vi "UDP Stream Reader.vi"() -> ()   [LabVIEW 2017]
uses:
  <vilib>/ptbypt/NI_PtbyPt.lvlib
panel:
  out "Chart":dbl(graph)=869191.9467676225
  out "Average Rate":dbl=904314.6721829617 format="%0.1pbytes/second"
  out "UDP Chunks Dropped":bool
  out "Total Heartbeats":i32=21
  out "Data Length":i32=17515
  in  "Stop":bool
  in  "Stream Source IP Address":string="localhost"
  # "UDP Streamer.vi must be running first!"
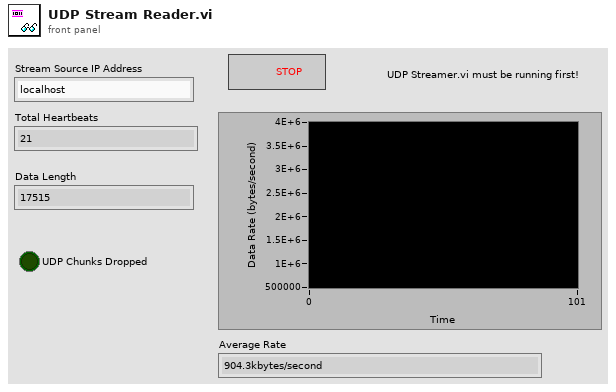
[diagram p1: front panel]
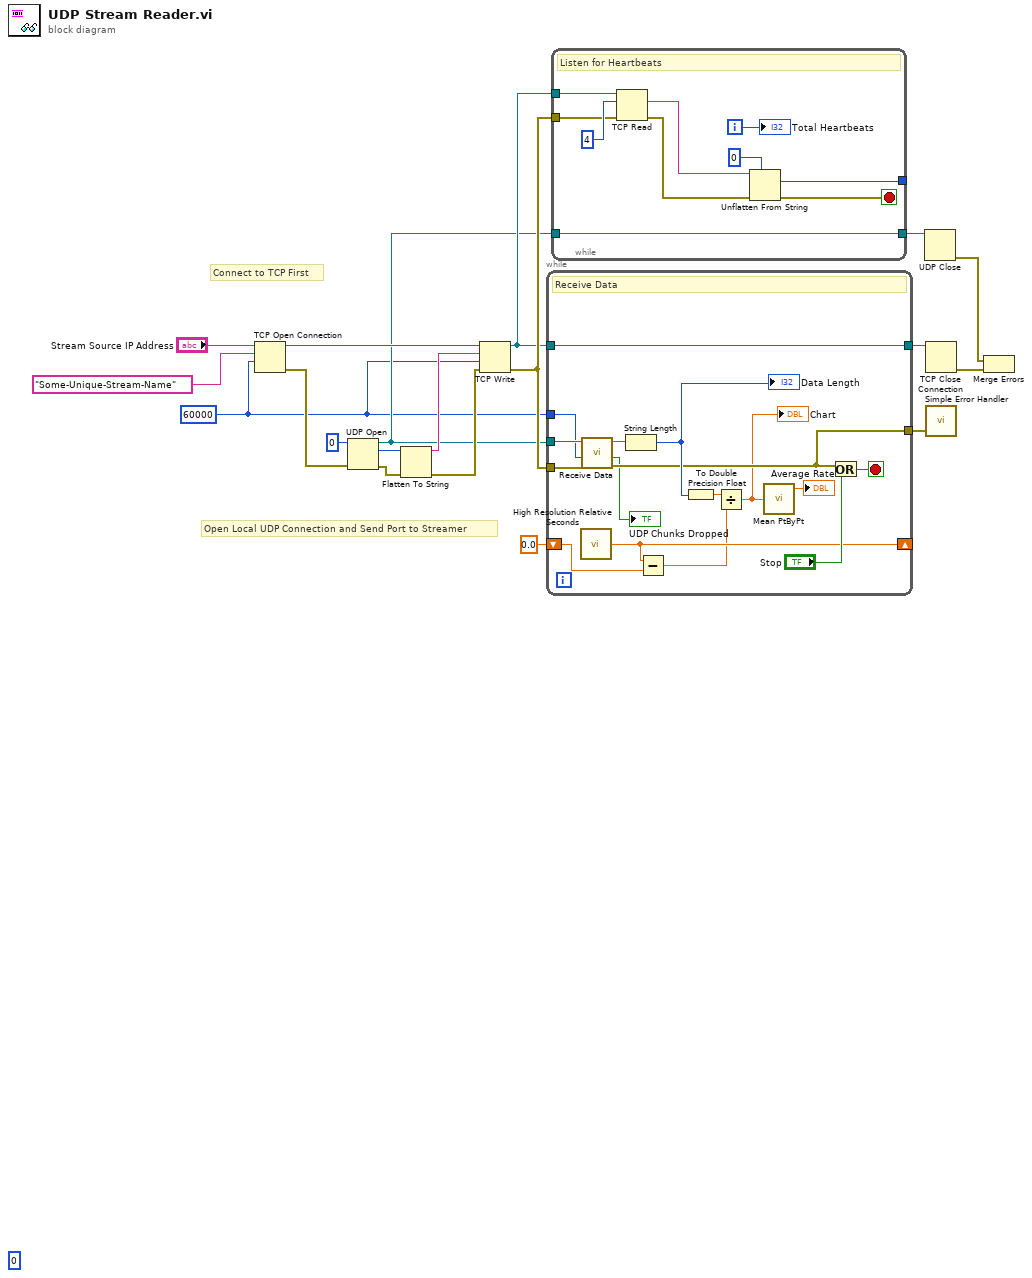
[diagram p0: block diagram]
diagram:
  w1 = 60000 ("timeout ms (60000)")
  (unwired) u32 0
  # "Open Local UDP Connection and Send Port to Streamer"
  # "Connect to TCP First"
  n1 = TCP Open Connection(address="Stream Source IP Address", remote port or service name="Some-Unique-Stream-Name", timeout ms (60000)=w1) -> (connection ID=w13:refnum<k5>, error out=w16:errorcluster)  [unwired: 2 in]
  n2 = UDP Open(8:w16, 11:u16 0 ("port")) -> (port=w7:refnum<k16>, 0:w15:errorcluster, 2:w14:u16)  [unwired: 3 in]
  n3 = Flatten To String(anything=w14, error in (no error)=w15) -> (data string=w11:string, error out=w12:errorcluster)  [unwired: 2 in, 1 out]
  n4 = TCP Write(connection ID=w13, data in=w11, error in (no error)=w12, 9:w1) -> (connection ID out=w8:refnum<k5>, error out=w10:errorcluster)  [unwired: 1 out]
  n5 = while {
    tunnel: w10 -> [w34]
    tunnel: [w33] -> w9
    tunnel: w8 -> [w33]
    tunnel: w7 -> [w35]
    shift-right: [w29] -> _
    shift-left: 0.0 ("relative seconds") -> [w30]
    tunnel: [w25] -> w2
    tunnel: w1 -> [w24]
    stop <- w31 stop-if-true
    # "Receive Data"
    n6 = call <vilib>:"High Resolution Relative Seconds.vi"() -> ("relative seconds"=w29:dbl)
    n7 = call "Receive Data.vi"("error in (no error)"=w34, "timeout ms (25000)"=w24, "UDP Network Connection in"=w35) -> ("error out"=w25:errorcluster, "Chunks Dropped"=→"UDP Chunks Dropped":bool, "Data"=w23:string)  [unwired: 6 in]
    n8 = String Length(string=w23) -> (length=w26:i32)
    "Data Length" <- w26
    n9 = Subtract(x=w29, y=w30) -> (x-y=w28:dbl)
    n10 = To Double Precision Float(number=w26) -> (double precision float=w27:dbl)
    n11 = Divide(x=w27, y=w28) -> (x/y=w20:dbl)
    "Chart" <- w20
    n12 = call <vilib>:"Mean PtByPt.vi"("x"=w20) -> ("mean"=→"Average Rate":dbl)  [unwired: 3 in, 1 out]
    n13 = Or(x=w25, y="Stop") -> (x .or. y?=w31:bool)
  }
  n14 = while {
    tunnel: w10 -> [w39]
    tunnel: w8 -> [w38]
    tunnel: w7 -> [w37]
    tunnel: [w37] -> w6
    tunnel: [w36] -> _
    i -> [w45]
    stop <- w40 stop-if-true
    # "Listen for Heartbeats"
    n15 = TCP Read(connection ID=w38, bytes to read=4, error in (no error)=w39) -> (data out=w43:string, error out=w41:errorcluster)  [unwired: 2 in, 1 out]
    n16 = Unflatten From String(type=0 ("bytes to read"), binary string=w43, error in (no error)=w41) -> (value=w36:i32, error out=w40:errorcluster)  [unwired: 2 in, 1 out]
    "Total Heartbeats" <- w45
  }
  n17 = UDP Close(connection ID=w6) -> (error out=w4:errorcluster)  [unwired: 1 in, 1 out]
  n18 = TCP Close Connection(connection ID=w9) -> (error out=w5:errorcluster)  [unwired: 2 in, 1 out]
  n19 = call <vilib>:"Simple Error Handler.vi"("error in (no error)"=w2) -> ()  [unwired: 4 in, 5 out]
  n20 = Merge Errors(w4, w5) -> ()  [unwired: 1 out]
